vi "reference-generator.vi"(8 "SamplingInt(s)":dbl, 9 "LockinPhase":dbl, 10 "LockinFreq":dbl, 11 "IntegrationPeriod(s)":dbl) -> (2 "Waveform Graph":waveform(dbl)[](graph), 3 "output cluster":cluster{dbl[], dbl[]})   [LabVIEW 2023]
doc: "Generates the Lock-In's reference signal."
uses:
  <vilib>/measure/NI_MABase.lvlib
  d16bb862-85c6-417e-9ce3-f8ddabda7635.vi
  8fe608f4-b201-43ca-ace0-678adbe8c443.vi
  6cbdd8f7-881a-47ab-b792-f3d13e9302af.vi
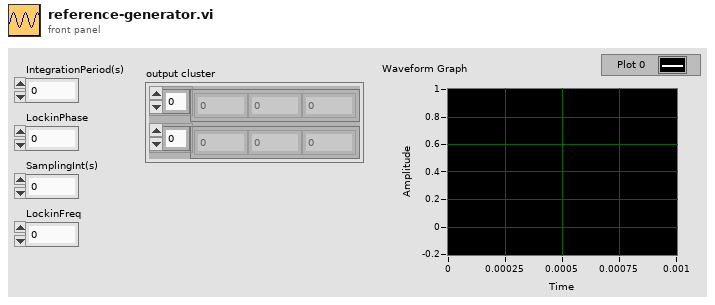
[diagram p1: front panel]
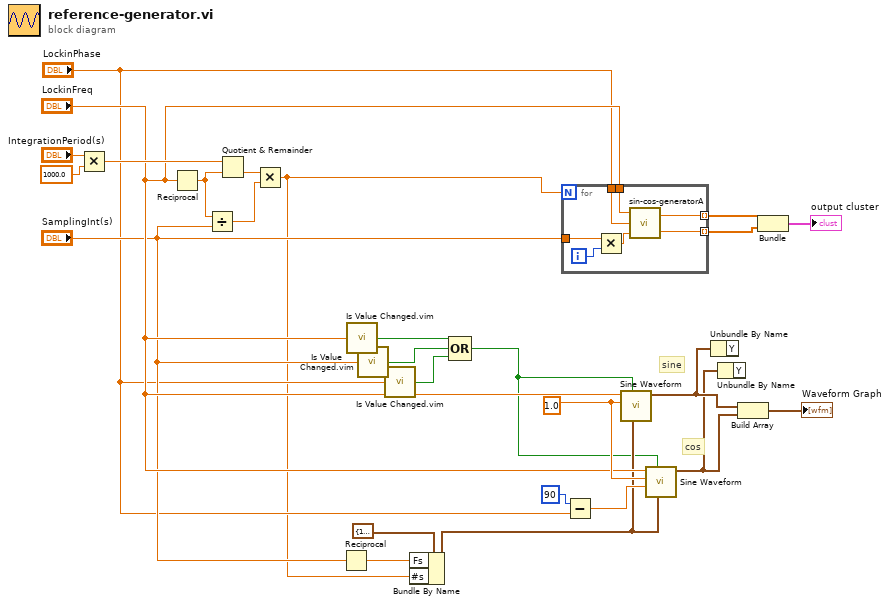
[diagram p0: block diagram]
diagram:
  w21 = 1.0 ("amplitude")
  # "cos"
  # "sine"
  n1 = Multiply(x="IntegrationPeriod(s)", y=1000.0) -> (x*y=w25:dbl)
  n2 = Reciprocal(x="LockinFreq") -> (1/x=w6:dbl)
  n3 = Divide(x=w6, y="SamplingInt(s)") -> (x/y=w8:dbl)
  n4 = Quotient & Remainder(x=w25, y=w6) -> (floor(x/y)=w7:dbl)  [unwired: 1 out]
  n5 = Multiply(x=w7, y=w8) -> (x*y=w3:dbl)
  n6 = Reciprocal(x="SamplingInt(s)") -> (1/x=w11:dbl)
  n7 = call "Is Value Changed.vim"("value"="LockinFreq") -> ("changed or first call?"=w17:bool)
  n8 = call "Is Value Changed.vim"("value"="SamplingInt(s)") -> ("changed or first call?"=w16:bool)
  n9 = call "Is Value Changed.vim"("value"="LockinPhase") -> ("changed or first call?"=w15:bool)
  n10 = Bundle By Name(cluster=cluster{"Fs":dbl, "#s":dbl} {"Fs"=1000.0, "#s"=1000.0} ("sampling info"), "Fs"=w11, "#s"=w3) -> (w18:cluster{"Fs":dbl, "#s":dbl})
  n11 = Compound Arithmetic op=OR(w17, w16, w15) -> (w14:bool)
  n12 = for {
    N: w3 -> [_]
    tunnel: "LockinPhase" -> [w33]
    tunnel: "LockinFreq" -> [w32]
    tunnel: "SamplingInt(s)" -> [w30]
    tunnel: [w28] -> w2 mode=indexing
    tunnel: [w27] -> w1 mode=indexing
    i -> [w31]
    n13 = Multiply(x=w30, y=w31) -> (x*y=w29:dbl)
    n14 = call "sin-cos-generatorA.vi"("Time"=w29, "Phase"=w33, "Frequency"=w32) -> ("cos"=w27:dbl, "sin"=w28:dbl)
  }
  n15 = Subtract(x=90, y="LockinPhase") -> (x-y=w22:dbl)
  n16 = call <vilib>:"Sine Waveform.vi"("sampling info"=w18, "reset signal"=w14, "amplitude"=w21, "frequency"="LockinFreq") -> ("signal out"=w5:waveform(dbl))  [unwired: 6 in, 1 out]
  n17 = call <vilib>:"Sine Waveform.vi"("sampling info"=w18, "reset signal"=w14, "phase"=w22, "amplitude"=w21, "frequency"="LockinFreq") -> ("signal out"=w4:waveform(dbl))  [unwired: 5 in, 1 out]
  n18 = Unbundle By Name(w5) -> ()  [unwired: 1 out]
  n19 = Unbundle By Name(w4) -> ()  [unwired: 1 out]
  n20 = Build Array(w5, w4) -> (→"Waveform Graph":waveform(dbl)[])
  n21 = Bundle(w2, w1) -> (→"output cluster":cluster{dbl[], dbl[]})  [unwired: 1 in]
